vi "Main_Sweep.vi"() -> ()   [LabVIEW 2016]
uses:
  Hardware/MW_ctl_Power_single..ctl
  Hardware/TrigerDelayer_ABCDEFGHDelay_ctl.ctl
  Hardware/TrigerDelayer_TriggerLevel&Source_ctl.ctl
  Hardware/TrigerDelayer_ctl_TriggerSource.ctl
  Main_Sweep_TemporaryVariable.ctl
  Main_Sweep_TemporaryVariable_Hardware.ctl
  Hardware/Hardware_DeviceAddresses.ctl
  Hardware/MW_ctl_DeviceHandles..ctl
  <instrlib>/Zurich Instruments LabOne/Public/ziTypeHandle.ctl
  <instrlib>/Zurich Instruments LabOne/Public/Modules/ziTypeModHandle.ctl
  Main_Sweep_TemporaryVariable_Data.ctl
  Hardware/MW_ctl_Souce Freq..ctl
  Hardware/Ctl_SetParameter(Value).ctl
  Hardware/MW_ctl_Powers.ctl
  <vilib>/Analysis/baseanly.llb/Mean (DBL).vi
  <instrlib>/Zurich Instruments LabOne/Public/Configure/ziSetValueDouble.vi
  <instrlib>/Zurich Instruments LabOne/Public/Modules/ziModSetValueBinaryArray.vi
  Hardware/HD_Device in Use(Array).vi
  <instrlib>/Zurich Instruments LabOne/Zurich Instruments LabOne.lvlib
  Hardware/ZI AWG.lvlib
  Hardware/General.lvlib
  Hardware/ZI LIA.lvlib
  Hardware/Microwave Source.lvlib
  Hardware/Trigger Delayer.lvlib
  <vilib>/Analysis/NI_AALBase.lvlib
panel:
  in  "Stop":bool
  in  "位置":dbl=0.5 step=0.1 format="%_3g"
  in  "Modulation Freq.":dbl=40000000.0 min=10.0 max=750000000.0 step=10000.0 format="%.3p"
  in  "Trigger Delayer Para.":T4
  in  "Tab Control":enum32{"MW Sweep", "AWG Sweep"}(tab)
  in  "LO":T5 {"Power dBm" min=-130.0 max=30.0 format="%.3p"}
  out "Current Freq(Hz) 2":dbl format="%#.6p"
  in  "Probe":T5 {"Power dBm" min=-130.0 max=30.0 format="%.3p"}
  out "Current Freq(Hz)":dbl format="%#.6p"
  in  "MW Sweep":bool
  in  "MW Sweep Parameters":T6={"Start"=4800000000.0, "Step"=10000000.0, "End"=9000000000.0, "Diff"=40000000.0} caption="Sweep Parameters" {"Diff" format="%.6pHZ"; "End" min=0.0 max=12000000000.0 step=100000000.0 format="%.6pHZ"; "Step" format="%.6pHZ"; "Start" min=0.0 max=12000000000.0 step=100000000.0 format="%.6pHZ"}
  out "Pulse Width":dbl min=0.0 max=40000.0 step=1.0 format="%#.3ps"
  out "AWG Points":cluster{"End":dbl, "Step":dbl, "Start":dbl} caption="Points" {"End" min=0.0 max=40000.0 step=1.0; "Start" min=0.0 max=12000000000.0 step=100000000.0}
  in  "AWG Sweep Parameters":cluster{"End":dbl, "Step":dbl, "Start":dbl}={"End"=1.5e-05, "Step"=2.0833e-08, "Start"=2e-07} caption="Sweep Parameters" {"End" min=1e-08 max=1.6e-05 step=1e-07 format="%#.3ps"; "Step" min=1e-09 max=1.5e-05 step=1e-08 format="%#.3ps"; "Start" min=2e-09 max=1.5e-05 step=1e-08 format="%#.3ps"}
  out "Reading":dbl min=0.0 max=40000.0 step=1.0 format="%.3p"
  in  "AWG Sweep":bool
  in  "Pulse Width":dbl=40000.0 min=0.0 max=40000.0 step=1.0 format="%.0f points"
  out "NULL Top":bool
  out "Devices in Use":string[][](table)
  out "error out":errorcluster
  out "DAQRead 耗时":u32
  in  "length":i32=10
  out "String":string
  out "size(s)":i32[](array[numeric])
  out "NULL Middle Left":bool
  out "NULL Middle Center":bool
  in  "ZoI Slide":cluster{i32, i32}(slide)={128, 155} scale=0.0..260.0
  out "ZoI Graph":dbl[][](graph)
  out "XY Graph":T7(graph)
  out "NULL Buttom Center 2":bool
  out "Demodulated R":dbl[][](graph)
  out "NULL Middle Right":bool
  out "Intensity Graph":dbl[][](graph)
  # "Local Oscillator"
  # "Probe"
  # "Debugging"
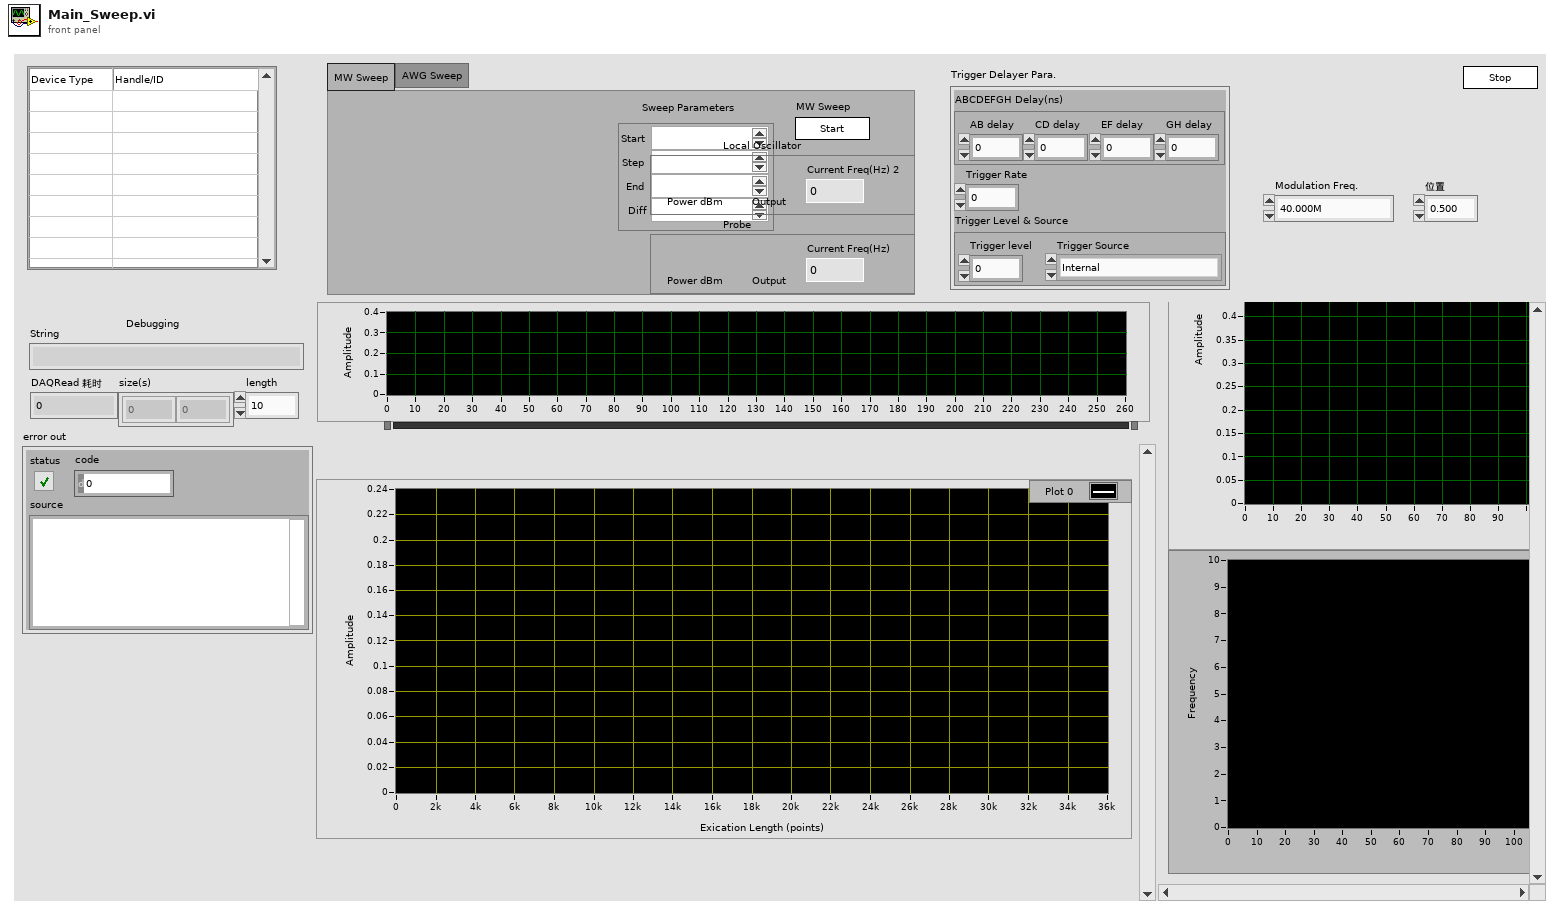
[diagram p1: front panel]
types:
  T1 = typedef "Trigger Delayer.lvlib/TrigerDelayer_ABCDEFGHDelay_ctl.ctl" = cluster{"AB delay":dbl, "CD delay":dbl, "EF delay":dbl, "GH delay":dbl}
  T2 = typedef "Trigger Delayer.lvlib/TrigerDelayer_TriggerLevel&Source_ctl.ctl" = cluster{"Trigger level":dbl, "Trigger Source":T3}
  T3 = typedef "Trigger Delayer.lvlib/TrigerDelayer_ctl_TriggerSource.ctl" = enum16{"Internal", "External Rising Edges", "External Falling Edges", "Single Shot External Rising Edges", "Single Shot External Falling Edges", "Single Shot", "Line"}
  T4 = cluster{"ABCDEFGH Delay(ns)":T1, "Trigger Rate":dbl, "Trigger Level & Source":T2}
  T5 = typedef "Microwave Source.lvlib/MW_ctl_Power_single..ctl" = cluster{"Output":bool, "Power dBm":dbl}
  T6 = cluster{"Start":dbl, "Step":dbl, "End":dbl, "Diff":dbl}
  T7 = cluster{"Sweep Para.":dbl[], "Sweep Readings":dbl[]}
  T8 = typedef "Main_Sweep_TemporaryVariable.ctl" = cluster{"Hardware Handle":T9, "Data":T14}
  T9 = typedef "Main_Sweep_TemporaryVariable_Hardware.ctl" = cluster{"Dev Add":T10, "AWG":T12, "LIA":T12, "LIA DAQ Mod":T13, "Devices in Use":string[][]}
  T10 = typedef "Hardware_DeviceAddresses.ctl" = cluster{"ZI Device Name":string[][], "MW Source":T11, "Trigger Delayer VISA":refnum<visa-resource-name>}
  T11 = typedef "Microwave Source.lvlib/MW_ctl_DeviceHandles..ctl" = cluster{"LO VISA":refnum<visa-resource-name>, "Probe VISA":refnum<visa-resource-name>, "Qubits":refnum<visa-resource-name>[]}
  T12 = typedef "Zurich Instruments LabOne.lvlib/ziTypeHandle.ctl" = cluster{"handleValid":bool, "Conn":u64, "Path Prefix":string, "Handle":u64, "Connected":bool, "Clockbase(s)":dbl}
  T13 = typedef "Zurich Instruments LabOne.lvlib/ziTypeModHandle.ctl" = cluster{"handleValid":bool, "Conn":u64, "ModHandle":u64, "moduleID":string, "Path Prefix":string}
  T14 = typedef "Main_Sweep_TemporaryVariable_Data.ctl" = cluster{"Demod R#1":dbl[][], "MW Source Freq":T15, "AWG PulseLength":cluster{"start":dbl, "step":dbl, "end":dbl, "iteration":dbl}, "Sweep Para.":cluster{"Sweep Para.":dbl[], "Sweep Readings":dbl[]}}
  T15 = typedef "Microwave Source.lvlib/MW_ctl_Souce Freq..ctl" = cluster{"start":dbl, "step":dbl, "end":dbl, "iteration":dbl, "diff":dbl}
  T16 = typedef "General.lvlib/Ctl_SetParameter(Value).ctl" = cluster{"Path":string, "Value":dbl, "comment":string}
  T17 = typedef "Microwave Source.lvlib/MW_ctl_Powers.ctl" = cluster{"LO":T5, "Probe":T5}
  T18 = cluster{"start":dbl, "step":dbl, "end":dbl, "iteration":dbl}
  T19 = typedef "LVRangeTypeDef.ctl" = cluster{"Minimum":dbl, "Maximum":dbl, "Increment":dbl, "Minor Increment":dbl, "Start":dbl}
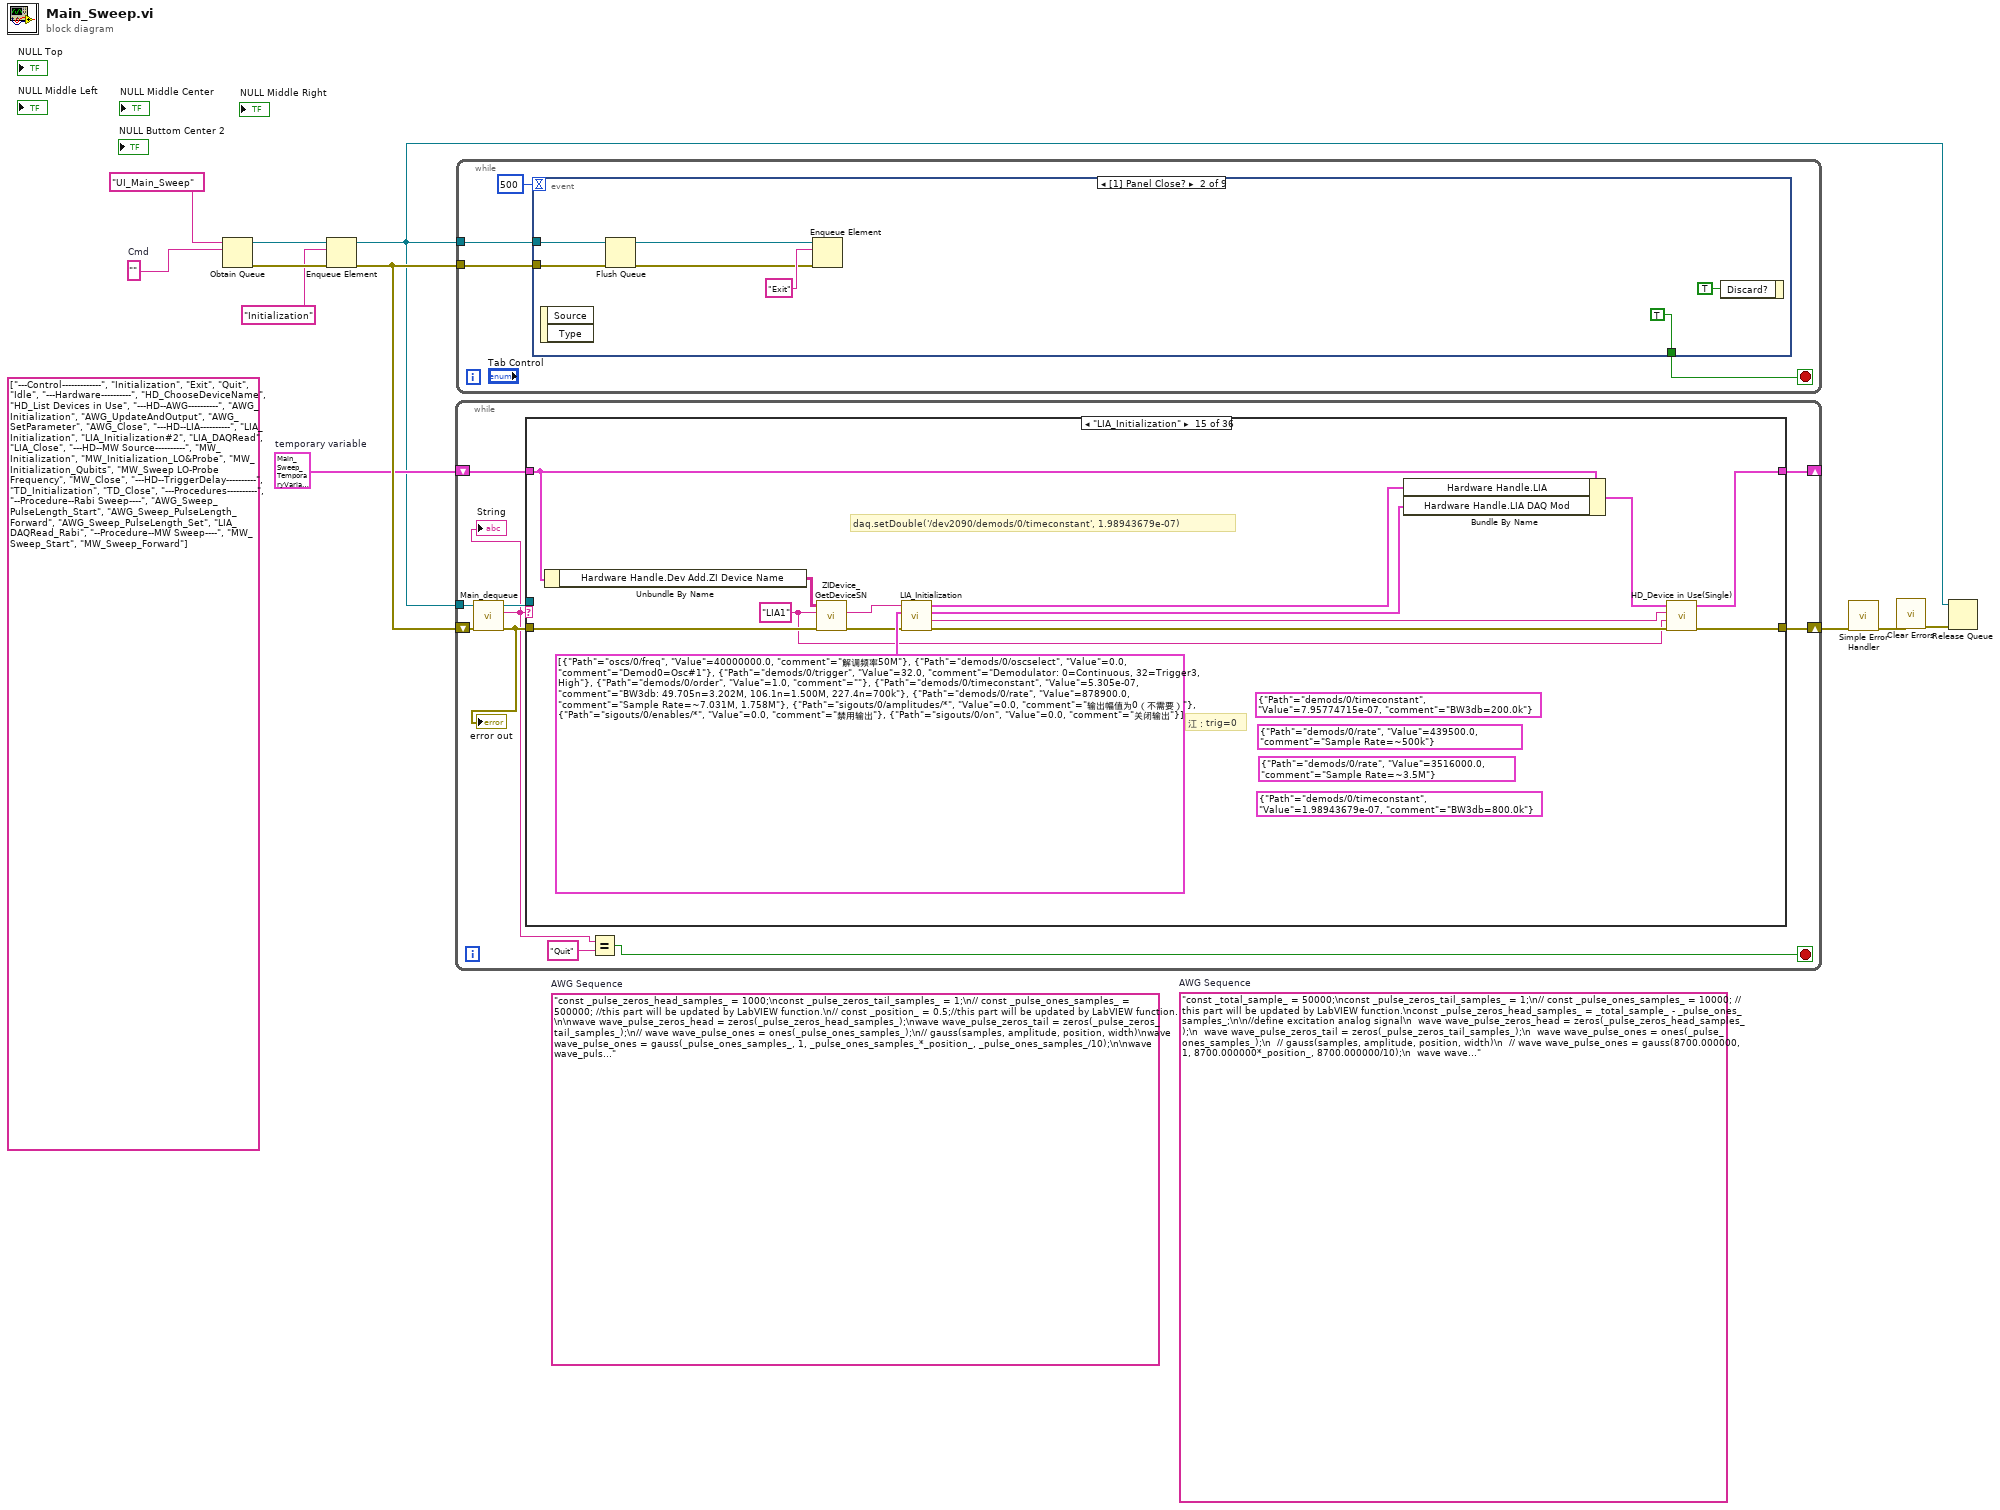
[diagram p0: block diagram]
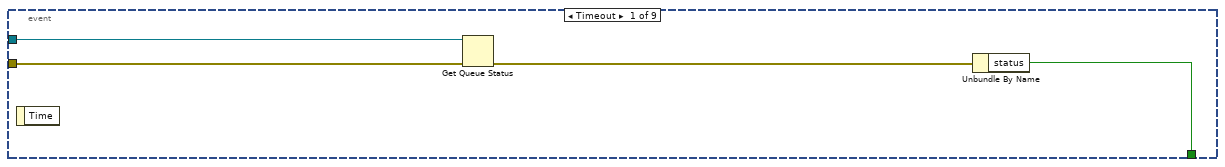
[diagram p2: hidden frame]
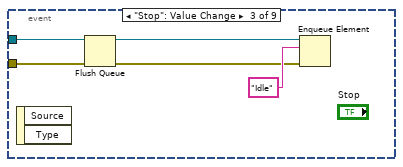
[diagram p3: hidden frame]
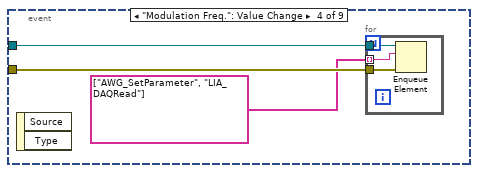
[diagram p4: hidden frame]
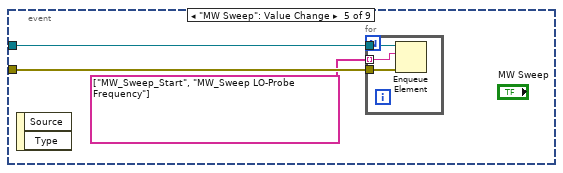
[diagram p5: hidden frame]
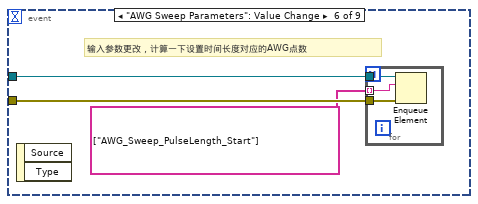
[diagram p6: hidden frame]
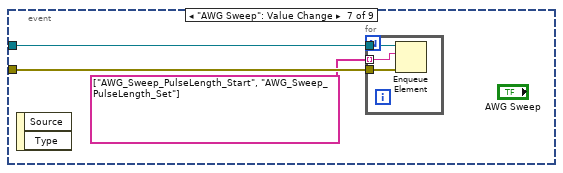
[diagram p7: hidden frame]
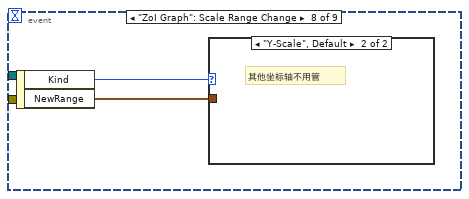
[diagram p8: hidden frame]
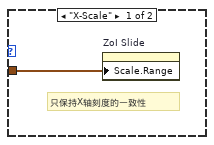
[diagram p9: hidden frame]
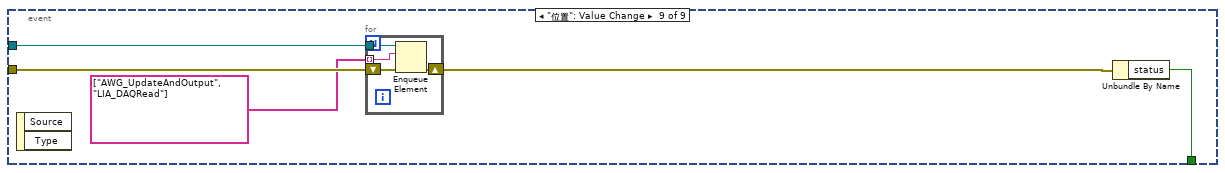
[diagram p10: hidden frame]
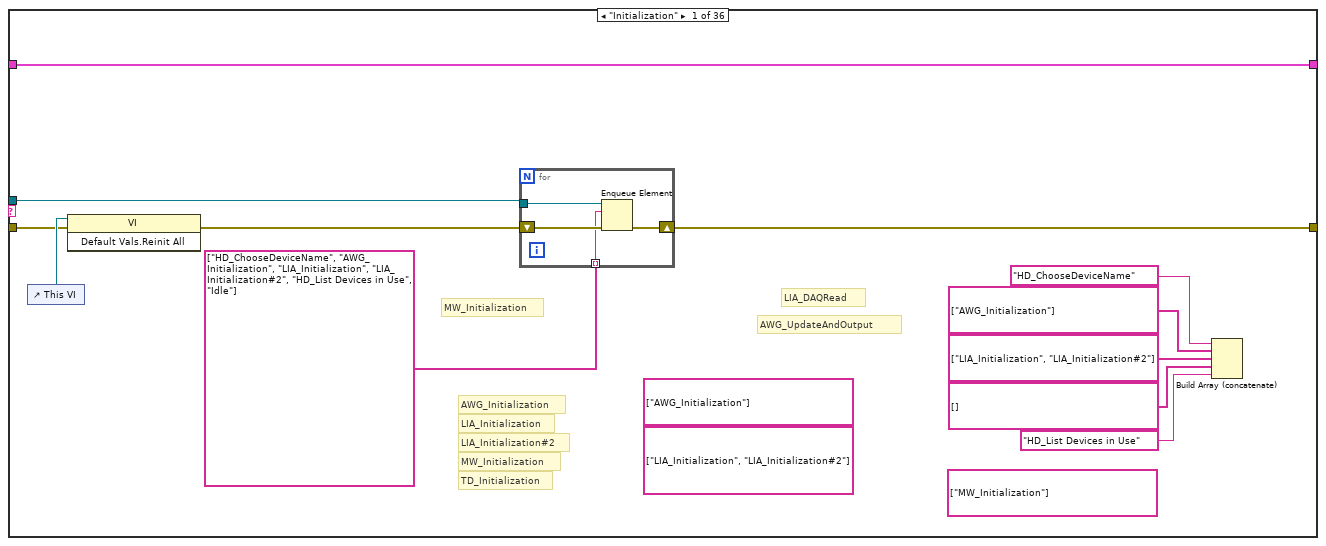
[diagram p11: hidden frame]
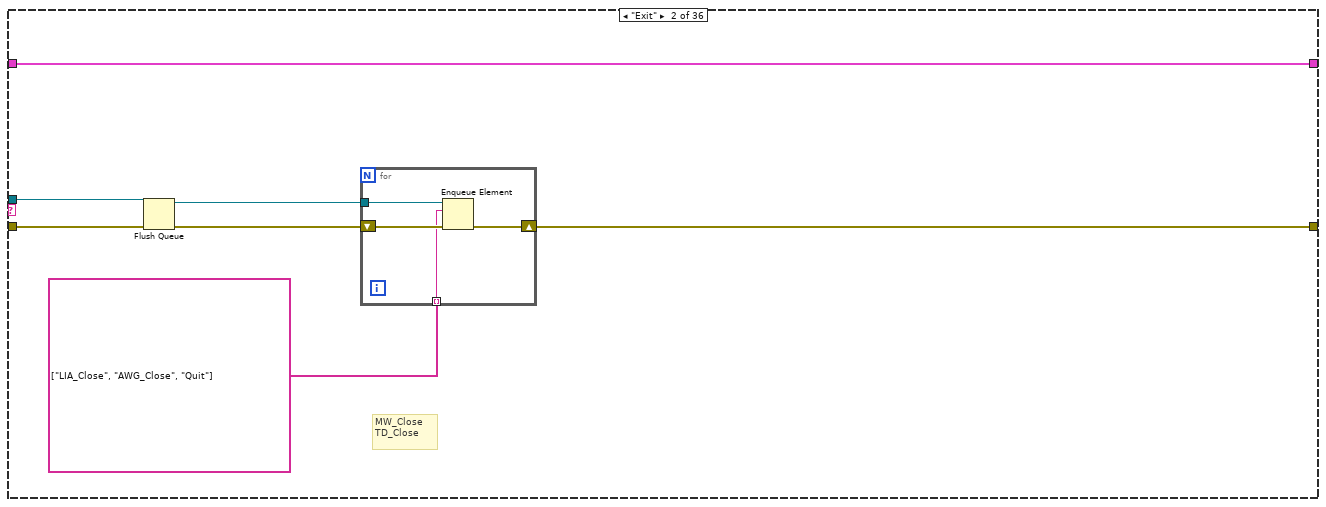
[diagram p12: hidden frame]
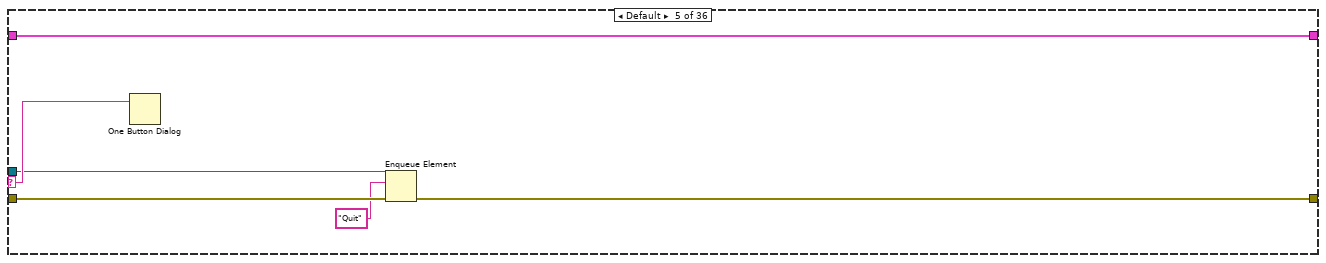
[diagram p15: hidden frame]
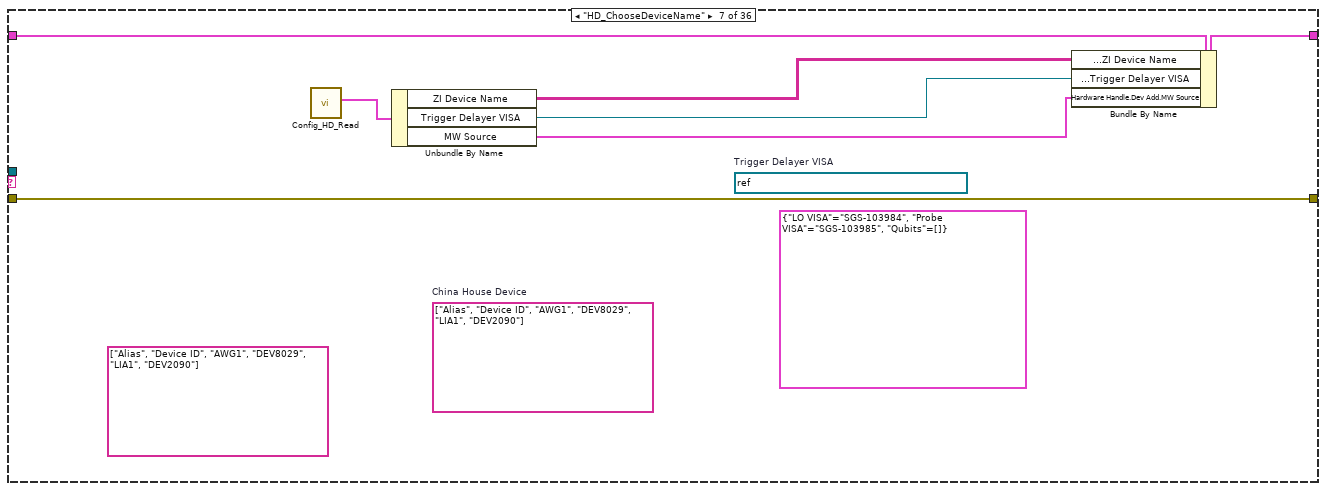
[diagram p17: hidden frame]
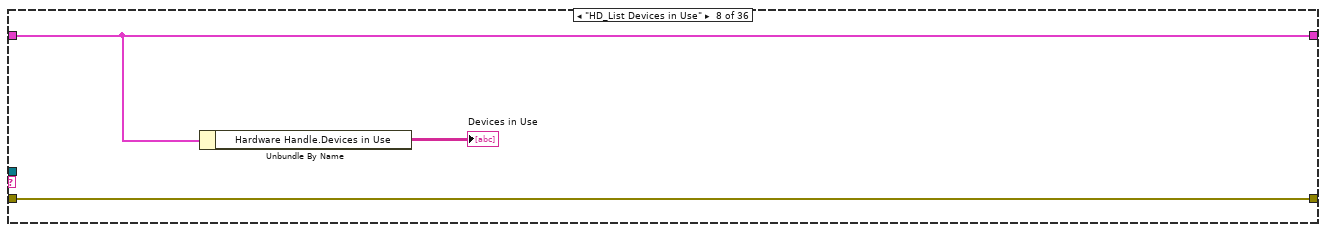
[diagram p18: hidden frame]
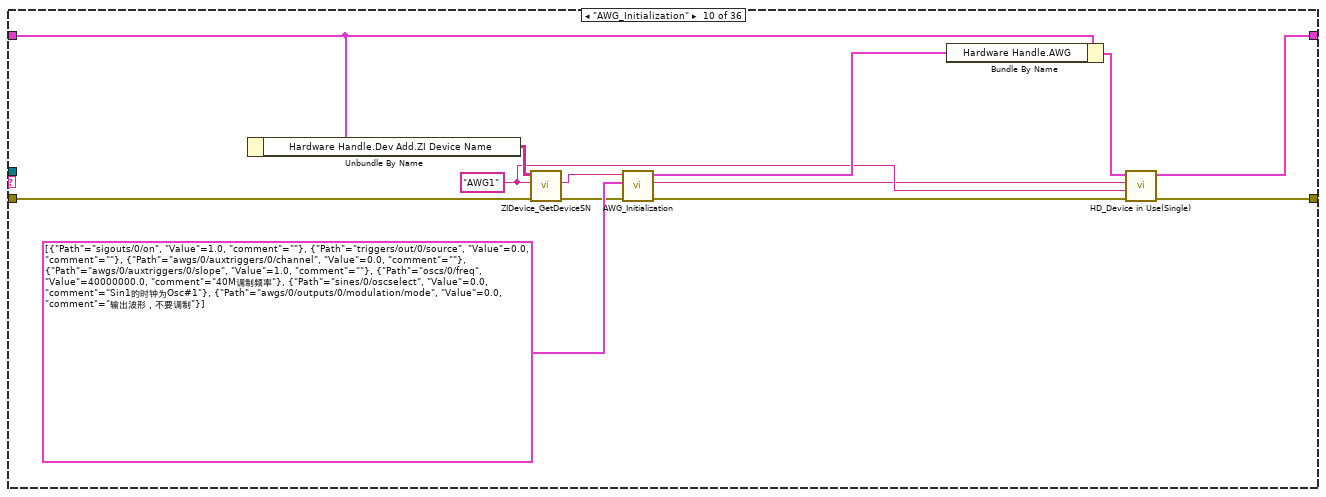
[diagram p20: hidden frame]
diagram:
  (unwired) "const _total_sample_ = 50000;\nconst _pulse_zeros_tail_samples_ = 1;\n// const _pulse_ones_samples_ = 10000; //this part will be updated by LabVIEW function.\nconst _pulse_zeros_head_samples_ = _total_sample_ - _pulse_ones_samples_;\n\n//define excitation analog signal\n  wave wave_pulse_zeros_head = zeros(_pulse_zeros_head_samples_);\n  wave wave_pulse_zeros_tail = zeros(_pulse_zeros_tail_samples_);\n  wave wave_pulse_ones = ones(_pulse_ones_samples_);\n  // gauss(samples, amplitude, position, width)\n  // wave wave_pulse_ones = gauss(8700.000000, 1, 8700.000000*_position_, 8700.000000/10);\n  wave wave_pulse = join(wave_pulse_zeros_head, wave_pulse_ones, wave_pulse_zeros_tail);\n//define marker\n  wave wave_marker_head = marker(10, 0);\n  wave wave_marker_ones = marker(_total_sample_-10*2, 1);\n  wave wave_marker_tail = marker(10, 0);\n  wave wave_mark = join(wave_marker_head, wave_marker_ones, wave_marker_tail);\n\nwave wave_output = wave_pulse + wave_mark;\n\nwhile (true){\n  waitDigTrigger(1); //External Trigger, to start AWG.\n  setTrigger(0b1111); // If you use \"AWG Trigger\" as DAQ read trigger, \"Mark out\" should be set to \"AWG Trigger 1\".\n  playWave(wave_output); //Alternative: Use \"Marker\" to trig DAQ read, \"Mark out\" should be set to \"Output 1 Marker 1\".\n  waitWave();\n  wait(500); //3.3ns per cycle.\n  setTrigger(0b0000);\n}"  # AWG Sequence
  (unwired) "const _pulse_zeros_head_samples_ = 1000;\nconst _pulse_zeros_tail_samples_ = 1;\n// const _pulse_ones_samples_ = 500000; //this part will be updated by LabVIEW function.\n// const _position_ = 0.5;//this part will be updated by LabVIEW function.\n\nwave wave_pulse_zeros_head = zeros(_pulse_zeros_head_samples_);\nwave wave_pulse_zeros_tail = zeros(_pulse_zeros_tail_samples_);\n// wave wave_pulse_ones = ones(_pulse_ones_samples_);\n// gauss(samples, amplitude, position, width)\nwave wave_pulse_ones = gauss(_pulse_ones_samples_, 1, _pulse_ones_samples_*_position_, _pulse_ones_samples_/10);\n\nwave wave_pulse = join(wave_pulse_zeros_head, wave_pulse_ones, wave_pulse_zeros_tail);\n\nwhile (true){\n  waitDigTrigger(1);\n  setTrigger(0b1111);\n  playWave(wave_pulse);\n  waitWave();\n  setTrigger(0b0000);\n}"  # AWG Sequence
  w5 = T8 {"Hardware Handle"={"Dev Add"={"ZI Device Name"=[], "MW Source"={"LO VISA"="", "Probe VISA"="", "Qubits"=[]}, "Trigger Delayer VISA"=""}, "AWG"={"handleValid"=FALSE, "Conn"=0, "Path Prefix"="", "Handle"=0, "Connected"=FALSE, "Clockbase(s)"=0.0}, "LIA"={"handleValid"=FALSE, "Conn"=0, "Path Prefix"="", "Handle"=0, "Connected"=FALSE, "Clockbase(s)"=0.0}, "LIA DAQ Mod"={"handleValid"=FALSE, "Conn"=0, "ModHandle"=0, "moduleID"="", "Path Prefix"=""}, "Devices in Use"=[]}, "Data"={"Demod R#1"=[], "MW Source Freq"={"start"=0.0, "step"=0.0, "end"=0.0, "iteration"=0.0, "diff"=0.0}, "AWG PulseLength"={"start"=0.0, "step"=0.0, "end"=0.0, "iteration"=0.0}, "Sweep Para."={"Sweep Para."=[], "Sweep Readings"=[]}}}  # temporary variable
  w11 = ""  # Cmd
  (unwired) string[] ["---Control-------------", "Initialization", "Exit", "Quit", "Idle", "---Hardware----------", "HD_ChooseDeviceName", "HD_List Devices in Use", "---HD--AWG----------", "AWG_Initialization", "AWG_UpdateAndOutput", "AWG_SetParameter", "AWG_Close", "---HD--LIA----------", "LIA_Initialization", "LIA_Initialization#2", "LIA_DAQRead", "LIA_Close", "---HD--MW Source----------", "MW_Initialization", "MW_Initialization_LO&Probe", "MW_Initialization_Qubits", "MW_Sweep LO-Probe Frequency", "MW_Close", "---HD--TriggerDelay----------", "TD_Initialization", "TD_Close", "---Procedures----------", "--Procedure--Rabi Sweep----", "AWG_Sweep_PulseLength_Start", "AWG_Sweep_PulseLength_Forward", "AWG_Sweep_PulseLength_Set", "LIA_DAQRead_Rabi", "--Procedure--MW Sweep----", "MW_Sweep_Start", "MW_Sweep_Forward"]
  n1 = Obtain Queue(name (unnamed)="UI_Main_Sweep", element data type=w11) -> (queue out=w9:refnum<queue>, error out=w8:errorcluster)  [unwired: 3 in, 1 out]
  n2 = Enqueue Element(queue=w9, element="Initialization", error in (no error)=w8) -> (queue out=w1:refnum<queue>, error out=w6:errorcluster)  [unwired: 1 in, 1 out]
  n3 = while {
    tunnel: w1 -> [w21]
    shift-right: [w18] -> _
    shift-left: w5 -> [w19]
    shift-right: [w14] -> w4
    shift-left: w6 -> [w20]
    stop <- w16 stop-if-true
    n4 = call "Main_dequeue.vi"("error in (no error)"=w20, "Queue in"=w21) -> ("error out"=w15:errorcluster, "Cmd"=w12:string, "Queue out"=w13:refnum<queue>)  [unwired: 7 in]
    "String" <- w12
    "error out" <- w15
    n5 = case shown="\"LIA_Initialization\"" w12 {
      selector: w12 -> [_ _ _ _ w57 _ _ _ _ _ _ _ _ _ _ _ _ _ _ _ _ _ _ _ _ _ _ _ _ _ _ _ _ _ _ _]
      tunnel: w19 -> [w31 w44 w50 w52 w58 w60 w66 w70 w72 w84 w103 w111 w117 w119 w133 w139 w168 w178 w180 w185 w203 w213 w245 w266 w270 w277 w292 w295 w297 w310 w318 w352 w367 w401 w412 w424]
      tunnel: [w31 w44 w50 w52 w58 w60 w65 w70 w72 w73 w100 w110 w116 w119 w120 w136 w167 w177 w180 w185 w194 w216 w252 w266 w270 w271 w292 w295 w297 w309 w333 w353 w359 w401 w411 w425] -> w18
      tunnel: w15 -> [w22 w40 w49 w51 w55 w59 w67 w68 w71 w80 w93 w109 w114 w118 w131 w142 w158 w172 w179 w182 w204 w214 w243 w268 w269 w279 w293 w294 w296 w303 w316 w345 w388 w400 w404 w417]
      tunnel: [w33 w43 w49 w51 w54 w59 w67 w68 w71 w77 w98 w108 w113 w118 w124 w144 w155 w175 w179 w181 w193 w215 w241 w267 w269 w276 w290 w294 w296 w302 w315 w346 w385 w400 w403 w418] -> w14
      tunnel: w13 -> [w32 w39 _ _ w56 _ _ _ _ _ _ _ _ _ _ _ _ _ _ w183 _ _ w251 _ _ _ _ _ _ _ w326 w343 _ _ _ w415]
      frame "Initialization" {
        (unwired) string[] ["LIA_Initialization", "LIA_Initialization#2"]
        (unwired) string[] ["AWG_Initialization"]
        (unwired) string[] ["MW_Initialization"]
        # "MW_Initialization"
        # "MW_Initialization"
        # "TD_Initialization"
        # "LIA_Initialization#2"
        # "LIA_Initialization"
        # "AWG_Initialization"
        # "AWG_UpdateAndOutput"
        # "LIA_DAQRead"
        n6 = control-ref of="This VI"() -> (w24:refnum<vi>)
        n7 = invoke class="VI" method="Default Vals.Reinit All"(reference=w24, error in=w22) -> (error out=w23:errorcluster)  [unwired: 1 in, 2 out]
        n8 = for {
          tunnel: string[] ["HD_ChooseDeviceName", "AWG_Initialization", "LIA_Initialization", "LIA_Initialization#2", "HD_List Devices in Use", "Idle"] -> [w35] mode=indexing
          tunnel: w32 -> [w34]
          shift-right: [w36] -> w33
          shift-left: w23 -> [w37]
          n9 = Enqueue Element(queue=w34, element=w35, error in (no error)=w37) -> (error out=w36:errorcluster)  [unwired: 1 in, 2 out]
        }
        n10 = Build Array (concatenate)("HD_ChooseDeviceName", string[] ["AWG_Initialization"], string[] ["LIA_Initialization", "LIA_Initialization#2"], string[] [], "HD_List Devices in Use") -> ()  [unwired: 1 out]
      }
      frame "Exit" {
        # "MW_Close\nTD_Close"
        n11 = Flush Queue(queue=w39, error in (no error)=w40) -> (queue out=w38:refnum<queue>, error out=w41:errorcluster)  [unwired: 1 out]
        n12 = for {
          tunnel: string[] ["LIA_Close", "AWG_Close", "Quit"] -> [w46] mode=indexing
          tunnel: w38 -> [w45]
          shift-right: [w47] -> w43
          shift-left: w41 -> [w48]
          n13 = Enqueue Element(queue=w45, element=w46, error in (no error)=w48) -> (error out=w47:errorcluster)  [unwired: 1 in, 2 out]
        }
      }
      frame "Quit" {
      }
      frame "Idle" {
      }
      frame Default {
        n14 = One Button Dialog(message=w57) -> ()  [unwired: 1 in, 1 out]
        n15 = Enqueue Element(queue=w56, element="Quit", error in (no error)=w55) -> (error out=w54:errorcluster)  [unwired: 1 in, 2 out]
      }
      frame "---Hardware----------" {
      }
      frame "HD_ChooseDeviceName" {
        (unwired) string[][] [["Alias", "Device ID"], ["AWG1", "DEV8029"], ["LIA1", "DEV2090"]]  # China House Device
        (unwired) refnum<visa-resource-name> "TCPIP0::192.168.2.10::5025::SOCKET"  # Trigger Delayer VISA
        (unwired) T11 {"LO VISA"="SGS-103984", "Probe VISA"="SGS-103985", "Qubits"=[]} ("MW Source In")
        (unwired) string[][] [["Alias", "Device ID"], ["AWG1", "DEV8029"], ["LIA1", "DEV2090"]] ("Hardware Handle.Device Name")
        n16 = call "Config_HD_Read.vi"() -> ("Dev Address"=w64:T10)  [unwired: 11 in]
        n17 = Unbundle By Name(w64) -> ("ZI Device Name"=w63:string[][], "Trigger Delayer VISA"=w62:refnum<visa-resource-name>, "MW Source"=w61:T11)
        n18 = Bundle By Name(cluster=w66, "Hardware Handle.Dev Add.ZI Device Name"=w63, "Hardware Handle.Dev Add.Trigger Delayer VISA"=w62, "Hardware Handle.Dev Add.MW Source"=w61) -> (w65:T8)
      }
      frame "HD_List Devices in Use" {
        n19 = Unbundle By Name(w70) -> ("Hardware Handle.Devices in Use"=→"Devices in Use":string[][])
      }
      frame "---HD--AWG----------" {
      }
      frame "AWG_Initialization" {
        w76 = "AWG1" ("alias")
        n20 = Unbundle By Name(w84) -> ("Hardware Handle.Dev Add.ZI Device Name"=w83:string[][])
        n21 = call "ZIDevice_GetDeviceSN.vi"("error in (no error)"=w80, "alias"=w76, "Hardware Handle.Device Name"=w83) -> ("error out"=w81:errorcluster, "Device SN"=w82:string)  [unwired: 7 in]
        n22 = call "AWG_Initialization.vi"("error in (no error)"=w81, "AWG Parameters"=T16[] [{"Path"="sigouts/0/on", "Value"=1.0, "comment"=""}, {"Path"="triggers/out/0/source", "Value"=0.0, "comment"=""}, {"Path"="awgs/0/auxtriggers/0/channel", "Value"=0.0, "comment"=""}, {"Path"="awgs/0/auxtriggers/0/slope", "Value"=1.0, "comment"=""}, {"Path"="oscs/0/freq", "Value"=40000000.0, "comment"="40M调制频率"}, {"Path"="sines/0/oscselect", "Value"=0.0, "comment"="Sin1的时钟为Osc#1"}, {"Path"="awgs/0/outputs/0/modulation/mode", "Value"=0.0, "comment"="输出波形，不要调制"}] ("Parameters"), "Address"=w82) -> ("error out"=w78:errorcluster, "Selected Device"=w75:string, "AWG Handle Out"=w79:T12)  [unwired: 6 in]
        n23 = Bundle By Name(cluster=w84, "Hardware Handle.AWG"=w79) -> (w74:T8)
        n24 = call "HD_Device in Use(Single).vi"("error in (no error)"=w78, "Alias"=w76, "Selected Device"=w75, "temporary variable In"=w74) -> ("error out"=w77:errorcluster, "temporary variable Out"=w73:T8)  [unwired: 6 in]
      }
      frame "AWG_UpdateAndOutput" {
        w94 = "const _pulse_zeros_tail_samples_ = 1;\n// const _pulse_ones_samples_ = 10000; //this part will be updated by LabVIEW function.\nconst _pulse_zeros_head_samples_ = 4000000 - _pulse_ones_samples_;\n\nwave wave_pulse_zeros_head = zeros(_pulse_zeros_head_samples_);\nwave wave_pulse_zeros_tail = zeros(_pulse_zeros_tail_samples_);\nwave wave_pulse_ones = ones(_pulse_ones_samples_);\n// gauss(samples, amplitude, position, width)\n// wave wave_pulse_ones = gauss(_pulse_ones_samples_, 1, _pulse_ones_samples_*_position_, _pulse_ones_samples_/10);\n\nwave wave_pulse = join(wave_pulse_zeros_head, wave_pulse_ones, wave_pulse_zeros_tail);\n\nwhile (true){\n  waitDigTrigger(1);\n  setTrigger(0b1111);\n  playWave(wave_pulse);\n  waitWave();\n  setTrigger(0b0000);\n}"  # AWG Sequence
        n25 = call "AWG_SequencyRewrite.vi"("error in (no error)"=w93, "Value"="Pulse Width", "Constant Name"="_pulse_ones_samples_", "AWG Sequence"=w94) -> ("error out"=w91:errorcluster, "result string"=w90:string)  [unwired: 5 in, 1 out]
        n26 = Unbundle By Name(w103) -> ("Hardware Handle.AWG"=w96:T12, "Hardware Handle.Dev Add.ZI Device Name"=w102:string[][])
        n27 = call "AWG_SequencyRewrite.vi"("Value"="位置", "Constant Name"="_position_", "AWG Sequence"=w90) -> ("result string"=w89:string)  [unwired: 6 in, 2 out]
        n28 = call "ZIDevice_GetDeviceSN.vi"("error in (no error)"=w91, "alias"="AWG1", "Hardware Handle.Device Name"=w102) -> ("error out"=w99:errorcluster, "Device SN"=w97:string)  [unwired: 7 in]
        n29 = call "AWG_UpdateWaveformAndOutput.vi"("Error In"=w99, "AWG Sequence"=w89, "Selected Device"=w97, "AWG Handle In"=w96) -> ("error out"=w98:errorcluster, "AWG Handle Out"=w95:T12)  [unwired: 6 in]
        n30 = Bundle By Name(cluster=w103, "Hardware Handle.AWG"=w95) -> (w100:T8)
      }
      frame "AWG_SetParameter" {
        w105 = "oscs/0/freq"  # 调制频率
        (unwired) T16 {"Path"="oscs/0/freq", "Value"=20000000.0, "comment"="20M调制频率"}
        n31 = Unbundle By Name(w111) -> ("Hardware Handle.AWG"=w107:T12)
        n32 = call-poly <instrlib>:"ziSetValue.vi"("Error In"=w109, "Value"="Modulation Freq.", "Path"=w105, "Handle In"=w107) -> ("Error Out"=w108:errorcluster, "Handle Out"=w106:T12)  [unwired: 1 in]
        n33 = Bundle By Name(cluster=w111, "Hardware Handle.AWG"=w106) -> (w110:T8)
      }
      frame "AWG_Close" {
        n34 = Unbundle By Name(w117) -> ("Hardware Handle.AWG"=w115:T12)
        n35 = call <instrlib>:"ziClose.vi"("Error In"=w114, "Handle In"=w115) -> ("Error Out"=w113:errorcluster, "Handle Out"=w112:T12)  [unwired: 2 in]
        n36 = Bundle By Name(cluster=w117, "Hardware Handle.AWG"=w112) -> (w116:T8)
      }
      frame "---HD--LIA----------" {
      }
      frame "LIA_Initialization" {
        (unwired) T16 {"Path"="demods/0/timeconstant", "Value"=1.98943679e-07, "comment"="BW3db=800.0k"}
        (unwired) T16 {"Path"="demods/0/rate", "Value"=3516000.0, "comment"="Sample Rate=~3.5M"}
        (unwired) T16 {"Path"="demods/0/rate", "Value"=439500.0, "comment"="Sample Rate=~500k"}
        (unwired) T16 {"Path"="demods/0/timeconstant", "Value"=7.95774715e-07, "comment"="BW3db=200.0k"}
        w123 = "LIA1" ("alias")
        # "daq.setDouble('/dev2090/demods/0/timeconstant', 1.98943679e-07)"
        # "江：trig=0"
        n37 = Unbundle By Name(w133) -> ("Hardware Handle.Dev Add.ZI Device Name"=w132:string[][])
        n38 = call "ZIDevice_GetDeviceSN.vi"("error in (no error)"=w131, "alias"=w123, "Hardware Handle.Device Name"=w132) -> ("error out"=w129:errorcluster, "Device SN"=w128:string)  [unwired: 7 in]
        n39 = call "LIA_Initialization.vi"("error in (no error)"=w129, "Lock-in Parameters"=T16[] [{"Path"="oscs/0/freq", "Value"=40000000.0, "comment"="解调频率50M"}, {"Path"="demods/0/oscselect", "Value"=0.0, "comment"="Demod0=Osc#1"}, {"Path"="demods/0/trigger", "Value"=32.0, "comment"="Demodulator: 0=Continuous, 32=Trigger3, High"}, {"Path"="demods/0/order", "Value"=1.0, "comment"=""}, {"Path"="demods/0/timeconstant", "Value"=5.305e-07, "comment"="BW3db: 49.705n=3.202M, 106.1n=1.500M, 227.4n=700k"}, {"Path"="demods/0/rate", "Value"=878900.0, "comment"="Sample Rate=~7.031M, 1.758M"}, {"Path"="sigouts/0/amplitudes/*", "Value"=0.0, "comment"="输出幅值为0（不需要）"}, {"Path"="sigouts/0/enables/*", "Value"=0.0, "comment"="禁用输出"}, {"Path"="sigouts/0/on", "Value"=0.0, "comment"="关闭输出"}], "Address"=w128) -> ("error out"=w125:errorcluster, "Selected Device"=w122:string, "DAQ ModHandle Out"=w126:T13, "Handle Out"=w127:T12)  [unwired: 5 in]
        n40 = Bundle By Name(cluster=w133, "Hardware Handle.LIA"=w127, "Hardware Handle.LIA DAQ Mod"=w126) -> (w121:T8)
        n41 = call "HD_Device in Use(Single).vi"("error in (no error)"=w125, "Alias"=w123, "Selected Device"=w122, "temporary variable In"=w121) -> ("error out"=w124:errorcluster, "temporary variable Out"=w120:T8)  [unwired: 6 in]
      }
      frame "LIA_Initialization#2" {
        w134 = "demods/0/sample.TrigIn3"  # Yuwei
        w147 = "/"
        (unwired) "demods/0/sample.TrigIn1"  # Dr. Jiang
        # "江：demods/0/sample.TrigIn1"
        n42 = Unbundle By Name(w139) -> ("Hardware Handle.LIA DAQ Mod"=w137:T13, "Hardware Handle.Dev Add.ZI Device Name"=w138:string[][])
        n43 = call "ZIDevice_GetDeviceSN.vi"("error in (no error)"=w142, "alias"="LIA1", "Hardware Handle.Device Name"=w138) -> ("error out"=w141:errorcluster, "Device SN"=w140:string)  [unwired: 7 in]
        n44 = Concatenate Strings(w147, w140, w147, w134) -> (w146:string)
        n45 = Build Array(w140, w146) -> (w151:string[])
        n46 = call-poly <instrlib>:"ziModSetValue.vi"("Error In"=w141, "Values"=w151, "Paths"=string[] ["dataAcquisitionModule/device", "dataAcquisitionModule/triggernode"], "ModHandle In"=w137) -> ("Error Out"=w148:errorcluster, "ModHandle Out"=w149:T13)  [unwired: 6 in]
        n47 = call "LIA_DAQ_SetModuleParameters.vi"("error in (no error)"=w148, "LIA DAQ Module Parameters"=T16[] [{"Path"="dataAcquisitionModule/delay", "Value"=0.0, "comment"="Delay(s)"}, {"Path"="dataAcquisitionModule/holdoff/time", "Value"=0.0001, "comment"="0.5ms内不再接受新触发"}, {"Path"="dataAcquisitionModule/holdoff/count", "Value"=0.0, "comment"=""}, {"Path"="dataAcquisitionModule/edge", "Value"=1.0, "comment"="上升沿触发"}, {"Path"="dataAcquisitionModule/grid/cols", "Value"=256.0, "comment"="Grid: 256 columns"}, {"Path"="dataAcquisitionModule/grid/rows", "Value"=100.0, "comment"="Rows: 至少为2！(推荐1k)"}, {"Path"="dataAcquisitionModule/endless", "Value"=0.0, "comment"="Single(单次运行)"}, {"Path"="dataAcquisitionModule/duration", "Value"=1e-05, "comment"=""}, {"Path"="dataAcquisitionModule/type", "Value"=1.0, "comment"="？？？？？"}, {"Path"="dataAcquisitionModule/historylength", "Value"=10.0, "comment"="历史长度10"}, {"Path"="dataAcquisitionModule/delay", "Value"=0.0, "comment"="Trigger position relative to"}, {"Path"="dataAcquisitionModule/type", "Value"=6.0, "comment"="触发类型：HW Trigger"}, {"Path"="dataAcquisitionModule/grid/mode", "Value"=4.0, "comment"="Exact(on-grid)"}], "DAQ ModHandle In"=w149) -> ("error out"=w144:errorcluster, "DAQ ModHandle Out"=w135:T13)  [unwired: 7 in]
        n48 = Bundle By Name(cluster=w139, "Hardware Handle.LIA DAQ Mod"=w135) -> (w136:T8)
      }
      frame "LIA_DAQRead" {
        w152 = 10  # History Length
        # "/dev2090/demods/0/sample.Theta.avg"
        n49 = Unbundle By Name(w168) -> ("Data.Sweep Para..Sweep Para."=w164:dbl[], "Data.Demod R#1"=w166:dbl[][], "Hardware Handle.LIA DAQ Mod"=w169:T13)
        n50 = local read "位置"() -> (w163:dbl)
        n51 = Build Array (concatenate)(w163, w164) -> (w162:dbl[])
        n52 = call "Tic Toc.vi"("error in (no error)"=w158) -> ("error out"=w157:errorcluster, "New Toc"=w154:u32)  [unwired: 8 in, 1 out]
        n53 = call "LIA_DAQ_Read.vi"("error in (no error)"=w157, "Subscribe Path Array"=string[] ["demods/0/sample.R"], "DAQ ModHandle In"=w169) -> ("error out"=w159:errorcluster, "Grid DEMOD R"=w160:dbl[][])  [unwired: 6 in, 1 out]
        n54 = call "calc_curve averaging.vi"("error in (no error)"=w159, "DAQ Read Array"=w160) -> ("error out"=w156:errorcluster, "Curve (Averaged)"=w153:dbl[])  [unwired: 7 in, 1 out]
        n55 = Build Array (concatenate)(w153, w166) -> (w165:dbl[][])
        n56 = call "Tic Toc.vi"("error in (no error)"=w156, "Last Tic"=w154) -> ("error out"=w155:errorcluster)  [unwired: 7 in, 2 out]
        n57 = Array Subset(array=w165, length (row)=w152) -> (w161:dbl[][])  [unwired: 3 in]
        n58 = Bundle By Name(cluster=w168, "Data.Sweep Para..Sweep Para."=w162, "Data.Demod R#1"=w161) -> (w167:T8)
      }
      frame "LIA_Close" {
        n59 = Unbundle By Name(w178) -> ("Hardware Handle.LIA"=w176:T12, "Hardware Handle.LIA DAQ Mod"=w171:T13)
        n60 = call <instrlib>:"ziModClear.vi"("Error In"=w172, "ziModHandle In"=w171) -> ("Error Out"=w173:errorcluster)  [unwired: 7 in, 1 out]
        n61 = call <instrlib>:"ziClose.vi"("Error In"=w173, "Handle In"=w176) -> ("Error Out"=w175:errorcluster, "Handle Out"=w174:T12)  [unwired: 2 in]
        n62 = Bundle By Name(cluster=w178, "Hardware Handle.LIA"=w174) -> (w177:T8)
      }
      frame "---HD--MW Source----------" {
      }
      frame "MW_Initialization" {
        n63 = for {
          tunnel: w183 -> [w189]
          tunnel: string[] ["MW_Initialization_LO&Probe", "MW_Initialization_Qubits"] -> [w187] mode=indexing
          shift-right: [w186] -> w181
          shift-left: w182 -> [w188]
          n64 = Enqueue Element At Opposite End(queue=w189, element=w187, error in (no error)=w188) -> (error out=w186:errorcluster)  [unwired: 1 in, 2 out]
        }
      }
      frame "MW_Initialization_LO&Probe" {
        n65 = Bundle By Name(cluster=T17 {"LO"={"Output"=FALSE, "Power dBm"=0.0}, "Probe"={"Output"=FALSE, "Power dBm"=0.0}} ("MW Power"), "LO"="LO", "Probe"="Probe") -> (w198:T17)
        n66 = Unbundle By Name(w203) -> ("Hardware Handle.Dev Add.MW Source"=w202:T11)
        n67 = call "MW_StartUp.vi"("error in (no error)"=w204, "MW Power"=w198, "MW Source In"=w202) -> ("error out"=w192:errorcluster, "MW Source Out"=w201:T11)  [unwired: 7 in]
        n68 = Bundle By Name(cluster=w203, "Hardware Handle.Dev Add.MW Source"=w201) -> (w195:T8)
        n69 = Unbundle By Name(w201) -> ("LO VISA"=w200:refnum<visa-resource-name>, "Probe VISA"=w199:refnum<visa-resource-name>)
        n70 = Build Array(w200, w199) -> (w191:refnum<visa-resource-name>[])
        n71 = call-poly "HD_Device in Use.vi"("error in (no error)"=w192, "Alias Array"=string[] ["MW LO", "MW Probe"], "Selected Devices Array"=w191, "temporary variable In"=w195) -> ("error out"=w193:errorcluster, "temporary variable Out"=w194:T8)  [unwired: 6 in]
      }
      frame "MW_Initialization_Qubits" {
        n72 = Unbundle By Name(w213) -> ("Hardware Handle.Dev Add.MW Source.Qubits"=w212:refnum<visa-resource-name>[])
        n73 = for {
          tunnel: 0.2 ("Delay Time (s)") -> [w231]
          tunnel: w212 -> [w230] mode=indexing
          shift-right: [w223] -> w209
          shift-left: w214 -> [w229]
          tunnel: T5[] [{"Output"=TRUE, "Power dBm"=0.0}, {"Output"=TRUE, "Power dBm"=0.0}] -> [w227] mode=indexing
          tunnel: [w224] -> w207 mode=indexing
          tunnel: dbl[] [4780000000.0] -> [w221] mode=indexing
          tunnel: [w217] -> w206 mode=indexing
          i -> [w220]
          n74 = VISA Open(error in (no error)=w229, VISA resource name=w230) -> (VISA resource name=w238:refnum<visa-resource-name>, error out=w237:errorcluster)  [unwired: 3 in]
          n75 = Unbundle By Name(w227) -> ("Power dBm"=w228:dbl)
          n76 = property class="Instr"(reference=w238, error in=w237, "General Settings:Timeout Value"=u32 125) -> (reference out=w235:refnum<visa-resource-name>, error out=w236:errorcluster)
          n77 = Format Into String(format string="%d", initial string="MW of Qubit #", w220) -> (resulting string=w217:string)  [unwired: 1 in, 1 out]
          n78 = call "MW_Set Power(dBm).vi"("错误输入（无错误）"=w236, "Power (dBm)"=w228, "VISA引用句柄输入"=w235) -> ("错误输出"=w232:errorcluster, "VISA引用句柄输出"=w234:refnum<visa-resource-name>)  [unwired: 6 in, 1 out]
          n79 = Unbundle By Name(w227) -> ("Output"=w226:bool)
          n80 = call "时间延迟"("error in (no error)"=w232, "Delay Time (s)"=w231) -> ("error out"=w233:errorcluster)  [unwired: 9 in]
          n81 = call "MW_Turn ON OFF.vi"("错误输入（无错误）"=w233, "start MW source?"=w226, "VISA引用句柄输入"=w234) -> ("错误输出"=w222:errorcluster, "VISA引用句柄输出"=w225:refnum<visa-resource-name>)  [unwired: 7 in]
          n82 = call "MW_Freq_Set and Confirm.vi"("错误输入（无错误）"=w222, "Set Frequency (Hz)"=w221, "VISA引用句柄输入"=w225) -> ("错误输出"=w223:errorcluster, "VISA引用句柄输出"=w224:refnum<visa-resource-name>)  [unwired: 6 in, 1 out]
        }
        n83 = call-poly "HD_Device in Use.vi"("error in (no error)"=w209, "Alias Array"=w206, "Selected Devices Array"=w207, "temporary variable In"=w213) -> ("error out"=w215:errorcluster, "temporary variable Out"=w216:T8)  [unwired: 6 in]
      }
      frame "MW_Sweep LO-Probe Frequency" {
        n84 = Unbundle By Name(w245) -> ("Data.MW Source Freq.start"=w249:dbl)
        n85 = Unbundle By Name(w245) -> ("Data.MW Source Freq.step"=w250:dbl, "Data.MW Source Freq.iteration"=w246:dbl)
        n86 = Unbundle By Name(w245) -> ("Data.MW Source Freq.diff"=w244:dbl)
        n87 = Multiply(x=w250, y=w246) -> (x*y=w248:dbl)
        n88 = Add(x=w249, y=w248) -> (x+y=w247:dbl)
        n89 = Unbundle By Name(w245) -> ("Hardware Handle.Dev Add.MW Source.LO VISA"=w259:refnum<visa-resource-name>)
        n90 = Unbundle By Name(w245) -> ("Hardware Handle.Dev Add.MW Source.Probe VISA"=w258:refnum<visa-resource-name>)
        n91 = Add(x=w247, y=w244) -> (x+y=w255:dbl)
        n92 = call "MW_Freq_Set and Confirm.vi"("错误输入（无错误）"=w243, "Set Frequency (Hz)"=w247, "VISA引用句柄输入"=w259) -> ("错误输出"=w260:errorcluster, "Current Freq(Hz)"=→"Current Freq(Hz) 2":dbl, "VISA引用句柄输出"=w254:refnum<visa-resource-name>)  [unwired: 6 in]
        n93 = call "MW_Freq_Set and Confirm.vi"("错误输入（无错误）"=w260, "Set Frequency (Hz)"=w255, "VISA引用句柄输入"=w258) -> ("错误输出"=w242:errorcluster, "Current Freq(Hz)"=→"Current Freq(Hz)":dbl, "VISA引用句柄输出"=w253:refnum<visa-resource-name>)  [unwired: 6 in]
        n94 = Bundle By Name(cluster=w245, "Hardware Handle.Dev Add.MW Source.LO VISA"=w254, "Hardware Handle.Dev Add.MW Source.Probe VISA"=w253) -> (w252:T8)
        n95 = for {
          tunnel: string[] ["LIA_DAQRead", "MW_Sweep_Forward"] -> [w264] mode=indexing
          tunnel: w251 -> [w263]
          shift-right: [w261] -> w241
          shift-left: w242 -> [w262]
          n96 = Enqueue Element(queue=w263, element=w264, error in (no error)=w262) -> (error out=w261:errorcluster)  [unwired: 1 in, 2 out]
        }
      }
      frame "MW_Close" {
        n97 = Unbundle By Name(w266) -> ("Hardware Handle.Dev Add.MW Source"=w265:T11)
        n98 = call "MW_Close.vi"("error in (no error)"=w268, "MW Source Out"=w265) -> ("error out"=w267:errorcluster)  [unwired: 9 in]
      }
      frame "---HD--TriggerDelay----------" {
      }
      frame "TD_Initialization" {
        n99 = Unbundle By Name(w277) -> ("Hardware Handle.Dev Add.Trigger Delayer VISA"=w278:refnum<visa-resource-name>)
        n100 = Unbundle By Name("Trigger Delayer Para.") -> ("Trigger Rate"=w283:dbl)
        n101 = VISA Open(error in (no error)=w279, VISA resource name=w278) -> (VISA resource name=w289:refnum<visa-resource-name>, error out=w288:errorcluster)  [unwired: 3 in]
        n102 = call "TrigerDelayer_TriggerRate_Set.vi"("error in (no error)"=w288, "Trigger Rate"=w283, "VISA Refnum in"=w289) -> ("error out"=w286:errorcluster, "VISA Refnum out"=w287:refnum<visa-resource-name>)  [unwired: 7 in]
        n103 = Unbundle By Name("Trigger Delayer Para.") -> ("Trigger Level & Source"=w282:T2)
        n104 = call "TrigerDelayer_TriggerLevel&Source_Set.vi"("error in (no error)"=w286, "Trigger Level & Source"=w282, "VISA Refnum in"=w287) -> ("error out"=w284:errorcluster, "VISA Refnum out"=w285:refnum<visa-resource-name>)  [unwired: 7 in]
        n105 = Unbundle By Name("Trigger Delayer Para.") -> ("ABCDEFGH Delay(ns)"=w280:T1)
        n106 = call "TrigerDelayer_ABCDEFGHDelay_Set.vi"("error in (no error)"=w284, "ABCDEFGH Delay(ns)"=w280, "VISA Refnum in"=w285) -> ("error out"=w275:errorcluster, "VISA Refnum out"=w273:refnum<visa-resource-name>)  [unwired: 7 in]
        n107 = Bundle By Name(cluster=w277, "Hardware Handle.Dev Add.Trigger Delayer VISA"=w273) -> (w272:T8)
        n108 = call "HD_Device in Use(Single).vi"("error in (no error)"=w275, "Alias"="Trigger Delayer", "Selected Device"=w273, "temporary variable In"=w272) -> ("error out"=w276:errorcluster, "temporary variable Out"=w271:T8)  [unwired: 6 in]
      }
      frame "TD_Close" {
        n109 = Unbundle By Name(w292) -> ("Hardware Handle.Dev Add.Trigger Delayer VISA"=w291:refnum<visa-resource-name>)
        n110 = VISA Close(VISA resource name=w291, error in (no error)=w293) -> (error out=w290:errorcluster)
      }
      frame "---Procedures----------" {
      }
      frame "--Procedure--Rabi Sweep----" {
      }
      frame "AWG_Sweep_PulseLength_Start" {
        w298 = 2400000000.0  # HDAWG Sample Rate
        w305 = 0.0  # start from zero
        n111 = property on="XY Graph" class="XYGraph (strict)"(error in=w303, "XScale.UnitLabel.Text"="Exication Length (points)" ("X Scale.Unit Label.Text")) -> (error out=w302:errorcluster)  [unwired: 1 in, 1 out]
        n112 = call "fun_TimeLength2Points(ClusterOfSweepPara).vi"("HDAWG Sample Rate (2.4GSa/s)"=w298, "AWG Sweep Parameters Time length (s)"="AWG Sweep Parameters") -> ("AWG Points"=w299:cluster{"End":dbl, "Step":dbl, "Start":dbl})  [unwired: 9 in]
        "AWG Points" <- w299
        n113 = Unbundle By Name(w299) -> ("Start"=w306:dbl, "Step"=w307:dbl, "End"=w308:dbl)
        n114 = Bundle By Name(cluster=w310, "Data.AWG PulseLength.start"=w306, "Data.AWG PulseLength.step"=w307, "Data.AWG PulseLength.end"=w308, "Data.AWG PulseLength.iteration"=w305, "Data.Sweep Para."=T7 {"Sweep Para."=[], "Sweep Readings"=[]}) -> (w309:T8)
      }
      frame "AWG_Sweep_PulseLength_Set" {
        w311 = "const _total_sample_ = 50000;\nconst _pulse_zeros_tail_samples_ = 1;\n// const _pulse_ones_samples_ = 10000; //this part will be updated by LabVIEW function.\nconst _pulse_zeros_head_samples_ = _total_sample_ - _pulse_ones_samples_;\n\n//define excitation analog signal\n  wave wave_pulse_zeros_head = zeros(_pulse_zeros_head_samples_);\n  wave wave_pulse_zeros_tail = zeros(_pulse_zeros_tail_samples_);\n  wave wave_pulse_ones = ones(_pulse_ones_samples_);\n  // gauss(samples, amplitude, position, width)\n  // wave wave_pulse_ones = gauss(8700.000000, 1, 8700.000000*_position_, 8700.000000/10);\n  wave wave_pulse = join(wave_pulse_zeros_head, wave_pulse_ones, wave_pulse_zeros_tail);\n//define marker\n  wave wave_marker_head = marker(_pulse_zeros_head_samples_, 0);\n  wave wave_marker_ones = marker(_pulse_ones_samples_, 1);\n  wave wave_marker_tail = marker(_pulse_zeros_tail_samples_, 0);\n  wave wave_mark = join(wave_marker_head, wave_marker_ones, wave_marker_tail);\n\nwave wave_output = wave_pulse + wave_mark;\n\nwhile (true){\n  waitDigTrigger(1); //External Trigger, to start AWG.\n  setTrigger(0b1111); // If you use \"AWG Trigger\" as DAQ read trigger, \"Mark out\" should be set to \"AWG Trigger 1\".\n  playWave(wave_output); //Alternative: Use \"Marker\" to trig DAQ read, \"Mark out\" should be set to \"Output 1 Marker 1\".\n  waitWave();\n  setTrigger(0b0000);\n  wait(500); //3.3ns per cycle.\n}"  # AWG Sequence
        w312 = 2400000000.0  # HDAWG Sample Rate
        (unwired) "const _total_sample_ = 50000;\nconst _pulse_zeros_tail_samples_ = 1;\n// const _pulse_ones_samples_ = 10000; //this part will be updated by LabVIEW function.\nconst _pulse_zeros_head_samples_ = _total_sample_ - _pulse_ones_samples_;\n\n//define excitation analog signal\n  wave wave_pulse_zeros_head = zeros(_pulse_zeros_head_samples_);\n  wave wave_pulse_zeros_tail = zeros(_pulse_zeros_tail_samples_);\n  wave wave_pulse_ones = ones(_pulse_ones_samples_);\n  // gauss(samples, amplitude, position, width)\n  // wave wave_pulse_ones = gauss(8700.000000, 1, 8700.000000*_position_, 8700.000000/10);\n  wave wave_pulse = join(wave_pulse_zeros_head, wave_pulse_ones, wave_pulse_zeros_tail);\n//define marker\n  wave wave_marker_head = marker(10, 0);\n  wave wave_marker_ones = marker(_total_sample_-10*2, 1);\n  wave wave_marker_tail = marker(10, 0);\n  wave wave_mark = join(wave_marker_head, wave_marker_ones, wave_marker_tail);\n\nwave wave_output = wave_pulse + wave_mark;\n\nwhile (true){\n  waitDigTrigger(1); //External Trigger, to start AWG.\n  setTrigger(0b1111); // If you use \"AWG Trigger\" as DAQ read trigger, \"Mark out\" should be set to \"AWG Trigger 1\".\n  playWave(wave_output); //Alternative: Use \"Marker\" to trig DAQ read, \"Mark out\" should be set to \"Output 1 Marker 1\".\n  waitWave();\n  wait(500); //3.3ns per cycle.\n  setTrigger(0b0000);\n}"  # AWG Sequence
        n115 = Unbundle By Name(w318) -> ("Data.AWG PulseLength"=w319:T18)
        n116 = Unbundle By Name(w319) -> ("start"=w322:dbl, "step"=w321:dbl, "iteration"=w320:dbl)
        n117 = for {
          tunnel: string[] ["LIA_DAQRead_Rabi", "AWG_Sweep_PulseLength_Forward"] -> [w339] mode=indexing
          tunnel: w326 -> [w338]
          shift-right: [w336] -> w317
          shift-left: w316 -> [w337]
          n118 = Enqueue Element(queue=w338, element=w339, error in (no error)=w337) -> (error out=w336:errorcluster)  [unwired: 1 in, 2 out]
        }
        n119 = Multiply(x=w321, y=w320) -> (x*y=w323:dbl)
        n120 = Add(x=w322, y=w323) -> (x+y=w314:dbl)
        n121 = call "fun_Points2TimeLength.vi"("HDAWG Sample Rate (2.4GSa/s)"=w312, "Points in AWG"=w314) -> ("Time Length (s)"=→"Pulse Width":dbl)  [unwired: 9 in]
        n122 = local write "Pulse Width"(w314) -> ()
        n123 = call "AWG_SequencyRewrite.vi"("error in (no error)"=w317, "Value"=w314, "Constant Name"="_pulse_ones_samples_", "AWG Sequence"=w311) -> ("error out"=w324:errorcluster, "result string"=w325:string)  [unwired: 5 in, 1 out]
        n124 = Unbundle By Name(w318) -> ("Hardware Handle.AWG"=w330:T12, "Hardware Handle.Dev Add.ZI Device Name"=w335:string[][])
        n125 = call "ZIDevice_GetDeviceSN.vi"("error in (no error)"=w324, "alias"="AWG1", "Hardware Handle.Device Name"=w335) -> ("error out"=w332:errorcluster, "Device SN"=w331:string)  [unwired: 7 in]
        n126 = call "AWG_UpdateWaveformAndOutput.vi"("Error In"=w332, "AWG Sequence"=w325, "Selected Device"=w331, "AWG Handle In"=w330) -> ("error out"=w315:errorcluster, "AWG Handle Out"=w329:T12)  [unwired: 6 in]
        n127 = Bundle By Name(cluster=w318, "Hardware Handle.AWG"=w329) -> (w333:T8)
      }
      frame "AWG_Sweep_PulseLength_Forward" {
        n128 = Unbundle By Name(w352) -> ("Data.AWG PulseLength.iteration"=w351:dbl)
        n129 = Increment(x=w351) -> (x+1=w350:dbl)
        n130 = Bundle By Name(cluster=w352, "Data.AWG PulseLength.iteration"=w350) -> (w353:T8)
        n131 = Unbundle By Name(w353) -> ("Data.AWG PulseLength"=w340:T18)
        n132 = Unbundle By Name(w340) -> ("start"=w356:dbl, "step"=w355:dbl, "iteration"=w354:dbl, "end"=w348:dbl)
        n133 = Multiply(x=w355, y=w354) -> (x*y=w357:dbl)
        n134 = Add(x=w356, y=w357) -> (x+y=w349:dbl)
        n135 = Greater Or Equal?(x=w349, y=w348) -> (x >= y?=w347:bool)
        n136 = Select(t="Idle" ("element"), s=w347, f="AWG_Sweep_PulseLength_Set" ("element")) -> (s? t:f=w344:string)
        n137 = Enqueue Element(queue=w343, element=w344, error in (no error)=w345) -> (error out=w346:errorcluster)  [unwired: 1 in, 2 out]
      }
      frame "LIA_DAQRead_Rabi" {
        # "/dev2090/demods/0/sample.Theta.avg"
        n138 = Unbundle By Name(w367) -> ("Data.Sweep Para..Sweep Para."=w365:dbl[], "Data.Sweep Para..Sweep Readings"=w362:dbl[], "Data.Demod R#1"=w397:dbl[][], "Hardware Handle.LIA DAQ Mod"=w398:T13)
        n139 = Unbundle By Name(w367) -> ("Data.AWG PulseLength"=w369:T18)
        n140 = call "Tic Toc.vi"("error in (no error)"=w388) -> ("error out"=w387:errorcluster, "New Toc"=w384:u32)  [unwired: 8 in, 1 out]
        n141 = Unbundle By Name(w369) -> ("start"=w371:dbl, "step"=w368:dbl, "iteration"=w370:dbl)
        n142 = call "LIA_DAQ_Read.vi"("error in (no error)"=w387, "Subscribe Path Array"=string[] ["demods/0/sample.R"], "DAQ ModHandle In"=w398) -> ("error out"=w389:errorcluster, "Grid DEMOD R"=w390:dbl[][])  [unwired: 6 in, 1 out]
        n143 = Multiply(x=w368, y=w370) -> (x*y=w372:dbl)
        n144 = call "calc_curve averaging.vi"("error in (no error)"=w389, "DAQ Read Array"=w390) -> ("error out"=w386:errorcluster, "Curve (Averaged)"=w376:dbl[])  [unwired: 7 in, 1 out]
        n145 = Add(x=w371, y=w372) -> (x+y=w366:dbl)
        n146 = Unbundle("ZoI Slide") -> (w377:i32, w382:i32)
        n147 = Build Array (concatenate)(w366, w365) -> (w364:dbl[])
        n148 = Subtract(x=w382, y=w377) -> (x-y=w381:i32)
        n149 = Build Array (concatenate)(w376, w397) -> (w396:dbl[][])
        n150 = call "Tic Toc.vi"("error in (no error)"=w386, "Last Tic"=w384) -> ("error out"=w385:errorcluster, "Consumed ticks"=→"DAQRead 耗时":u32)  [unwired: 7 in, 1 out]
        n151 = Array Size(array=w376) -> (size(s)=w380:i32)
        n152 = Array Subset(array=w376, index=w377, length=w381) -> (w363:dbl[])
        n153 = Initialize Array(-inf, w380) -> (w378:dbl[])
        n154 = Replace Array Subset(array=w378, new element=w363, index=w377) -> (w375:dbl[])
        n155 = call-poly <vilib>:"Mean.vi"("X"=w363) -> ("mean"=w360:dbl)  [unwired: 1 out]
        "Reading" <- w360
        n156 = Build Array(w376, w375) -> (→"ZoI Graph":dbl[][])
        n157 = Build Array (concatenate)(w360, w362) -> (w361:dbl[])
        n158 = Array Subset(array=w396, length (row)="length") -> (w391:dbl[][])  [unwired: 3 in]
        "Demodulated R" <- w391
        n159 = Bundle By Name(cluster=w367, "Data.Sweep Para..Sweep Para."=w364, "Data.Sweep Para..Sweep Readings"=w361, "Data.Demod R#1"=w391) -> (w359:T8)
        n160 = Transpose 2D Array(2D array=w391) -> (transposed array=w393:dbl[][])
        n161 = Array Size(array=w391) -> (size(s)=→"size(s)":i32[])
        n162 = Logarithm Base 10(1:w393) -> (0:→"Intensity Graph":dbl[][])
        n163 = Unbundle By Name(w359) -> ("Data.Sweep Para."=→"XY Graph":T7)
      }
      frame "--Procedure--MW Sweep----" {
      }
      frame "MW_Sweep_Start" {
        w410 = 0.0  # start from zero
        n164 = Unbundle By Name("MW Sweep Parameters") -> ("Start"=w405:dbl, "Step"=w406:dbl, "End"=w407:dbl, "Diff"=w408:dbl)
        n165 = property on="XY Graph" class="XYGraph (strict)"(error in=w404, "XScale.UnitLabel.Text"="Frequency (Hz)" ("X Scale.Unit Label.Text")) -> (error out=w403:errorcluster)  [unwired: 1 in, 1 out]
        n166 = Bundle By Name(cluster=w412, "Data.MW Source Freq.start"=w405, "Data.MW Source Freq.step"=w406, "Data.MW Source Freq.end"=w407, "Data.MW Source Freq.diff"=w408, "Data.MW Source Freq.iteration"=w410) -> (w411:T8)
      }
      frame "MW_Sweep_Forward" {
        n167 = Unbundle By Name(w424) -> ("Data.MW Source Freq.iteration"=w423:dbl)
        n168 = Increment(x=w423) -> (x+1=w422:dbl)
        n169 = Bundle By Name(cluster=w424, "Data.MW Source Freq.iteration"=w422) -> (w425:T8)
        n170 = Unbundle By Name(w425) -> ("Data.MW Source Freq.start"=w428:dbl, "Data.MW Source Freq.step"=w427:dbl, "Data.MW Source Freq.iteration"=w426:dbl, "Data.MW Source Freq.end"=w420:dbl)
        n171 = Multiply(x=w427, y=w426) -> (x*y=w429:dbl)
        n172 = Add(x=w428, y=w429) -> (x+y=w421:dbl)
        n173 = Greater Or Equal?(x=w421, y=w420) -> (x >= y?=w419:bool)
        n174 = Select(t="Idle" ("element"), s=w419, f="MW_Sweep LO-Probe Frequency" ("element")) -> (s? t:f=w416:string)
        n175 = Enqueue Element(queue=w415, element=w416, error in (no error)=w417) -> (error out=w418:errorcluster)  [unwired: 1 in, 2 out]
      }
    }
    n176 = Equal?(x=w12, y="Quit") -> (x = y?=w16:bool)
  }
  n177 = while {
    tunnel: w1 -> [w433]
    tunnel: w6 -> [w432]
    stop <- w431 stop-if-true
    n178 = event shown="[1] Panel Close?" {
      selector: _ -> [_ _ _ _ _ _ _ _ _]
      dyn-events: _ -> [_ _ _ _ _ _ _ _ _]
      timeout: 500 -> [_ _ _ _ _ _ _ _ _]
      tunnel: w433 -> [w434 w442 w449 w452 w458 w464 w470 _ w481]
      tunnel: w432 -> [w437 w438 w445 w451 w457 w463 w469 _ w480]
      tunnel: [w436 TRUE _ _ _ _ _ _ w477] -> w431
      event Timeout {
        n179 = event-data() -> ()  [unwired: 1 in, 1 out]
        n180 = Get Queue Status(queue=w434, error in (no error)=w437) -> (error out=w435:errorcluster)  [unwired: 1 in, 7 out]
        n181 = Unbundle By Name(w435) -> ("status"=w436:bool)
      }
      event Panel Close? {
        n182 = event-data() -> ()  [unwired: 1 in, 2 out]
        n183 = Flush Queue(queue=w442, error in (no error)=w438) -> (queue out=w440:refnum<queue>, error out=w439:errorcluster)  [unwired: 1 out]
        n184 = Enqueue Element(queue=w440, element="Exit", error in (no error)=w439) -> ()  [unwired: 1 in, 3 out]
        n185 = event-data("Discard?"=TRUE) -> ()  [unwired: 1 in, 1 out]
      }
      event "Stop": Value Change {
        n186 = event-data() -> ()  [unwired: 1 in, 2 out]
        n187 = Flush Queue(queue=w449, error in (no error)=w445) -> (queue out=w447:refnum<queue>, error out=w446:errorcluster)  [unwired: 1 out]
        n188 = Enqueue Element(queue=w447, element="Idle", error in (no error)=w446) -> ()  [unwired: 1 in, 3 out]
      }
      event "Modulation Freq.": Value Change {
        n189 = event-data() -> ()  [unwired: 1 in, 2 out]
        n190 = for {
          tunnel: w452 -> [w455]
          tunnel: w451 -> [w454]
          tunnel: string[] ["AWG_SetParameter", "LIA_DAQRead"] -> [w453] mode=indexing
          n191 = Enqueue Element(queue=w455, element=w453, error in (no error)=w454) -> ()  [unwired: 1 in, 3 out]
        }
      }
      event "MW Sweep": Value Change {
        n192 = event-data() -> ()  [unwired: 1 in, 2 out]
        n193 = for {
          tunnel: w458 -> [w461]
          tunnel: w457 -> [w460]
          tunnel: string[] ["MW_Sweep_Start", "MW_Sweep LO-Probe Frequency"] -> [w459] mode=indexing
          n194 = Enqueue Element(queue=w461, element=w459, error in (no error)=w460) -> ()  [unwired: 1 in, 3 out]
        }
      }
      event "AWG Sweep Parameters": Value Change {
        # "输入参数更改，计算一下设置时间长度对应的AWG点数"
        n195 = event-data() -> ()  [unwired: 1 in, 2 out]
        n196 = for {
          tunnel: w464 -> [w467]
          tunnel: w463 -> [w466]
          tunnel: string[] ["AWG_Sweep_PulseLength_Start"] -> [w465] mode=indexing
          n197 = Enqueue Element(queue=w467, element=w465, error in (no error)=w466) -> ()  [unwired: 1 in, 3 out]
        }
      }
      event "AWG Sweep": Value Change {
        n198 = event-data() -> ()  [unwired: 1 in, 2 out]
        n199 = for {
          tunnel: w470 -> [w473]
          tunnel: w469 -> [w472]
          tunnel: string[] ["AWG_Sweep_PulseLength_Start", "AWG_Sweep_PulseLength_Set"] -> [w471] mode=indexing
          n200 = Enqueue Element(queue=w473, element=w471, error in (no error)=w472) -> ()  [unwired: 1 in, 3 out]
        }
      }
      event "ZoI Graph": Scale Range Change {
        n201 = event-data() -> ("Kind"=w474:enum16{"X-Scale", "Y-Scale", "Z-Scale"}, "NewRange"=w475:T19)  [unwired: 1 in]
        n202 = case shown="\"Y-Scale\", Default" w474 {
          tunnel: w475 -> [w476 _]
          frame "X-Scale" {
            # "只保持X轴刻度的一致性"
            n203 = property on="ZoI Slide" class="Slide (strict)"("Scale.Range"=w476) -> ()  [unwired: 2 in, 2 out]
          }
          frame "Y-Scale", Default {
            # "其他坐标轴不用管"
          }
        }
      }
      event "位置": Value Change {
        n204 = event-data() -> ()  [unwired: 1 in, 2 out]
        n205 = for {
          tunnel: w481 -> [w485]
          tunnel: string[] ["AWG_UpdateAndOutput", "LIA_DAQRead"] -> [w483] mode=indexing
          shift-right: [w482] -> w478
          shift-left: w480 -> [w484]
          n206 = Enqueue Element(queue=w485, element=w483, error in (no error)=w484) -> (error out=w482:errorcluster)  [unwired: 1 in, 2 out]
        }
        n207 = Unbundle By Name(w478) -> ("status"=w477:bool)
      }
    }
  }
  n208 = call <vilib>:"Simple Error Handler.vi"("error in (no error)"=w4) -> ("error out"=w3:errorcluster)  [unwired: 4 in, 4 out]
  n209 = call <vilib>:"Clear Errors.vi"("error in (no error)"=w3) -> ("error out"=w2:errorcluster)  [unwired: 5 in, 1 out]
  n210 = Release Queue(queue=w1, error in (no error)=w2) -> ()  [unwired: 1 in, 3 out]
